vi "DSF.Engine.Memory.Buffer.Check.vi"(8 "error in (no error)":errorcluster, 11 "Buffer in":refnum<class "DSF.Engine.Memory.Buffer.lvclass">) -> (0 "error out":errorcluster, 3 "Buffer out":refnum<class "DSF.Engine.Memory.Buffer.lvclass">)   [LabVIEW 2016, in "DSF.Engine.lvlib" / "DSF.Engine.Memory.Buffer.lvclass"]
uses:
  DSF.Engine.Memory.Buffer.lvclass
  DSF.Engine.Memory.Buffer.lvclass/DSF.Engine.Memory.Buffer.ctl
  DSF.Engine.Memory.Buffer.Errors.Invalid Buffer.vi
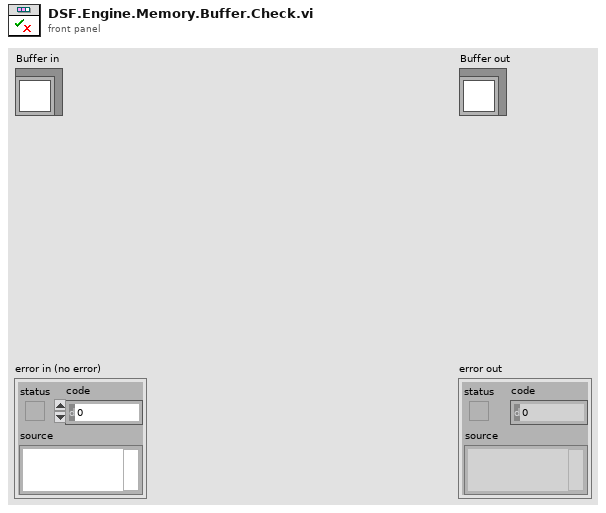
[diagram p1: front panel]
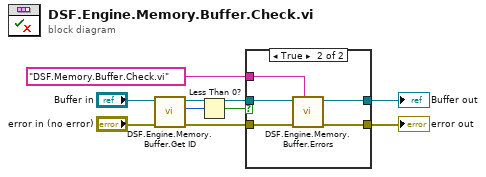
[diagram p0: block diagram]
diagram:
  n1 = call "DSF.Engine.Memory.Buffer.Get ID.vi"("error in (no error)"="error in (no error)", "Buffer in"="Buffer in") -> ("error out"=w6:errorcluster, "id"=w7:i32, "Buffer out"=w5:refnum<class "DSF.Engine.Memory.Buffer.lvclass">)  [unwired: 7 in]
  n2 = Less Than 0?(x=w7) -> (x < 0?=w4:bool)
  n3 = case shown="True" w4 {
    tunnel: w6 -> [w10 w15]
    tunnel: w5 -> [w11 w16]
    tunnel: [w11 w14] -> w2
    tunnel: [w10 w13] -> w3
    tunnel: "DSF.Memory.Buffer.Check.vi" ("calling vi name") -> [_ w12]
    frame False {
    }
    frame True {
      n4 = call-poly "DSF.Engine.Memory.Buffer.Errors.vi"("calling vi name"=w12, "error in (no error)"=w15, "Buffer in"=w16) -> ("error out"=w13:errorcluster, "Buffer out"=w14:refnum<class "DSF.Engine.Memory.Buffer.lvclass">)  [unwired: 7 in]
    }
  }
  "error out" <- w3
  "Buffer out" <- w2
